vi "Write Calibration File.vi"(6 "CalDataIn":T1(array[cluster]) {"ChlFactor" format="%.3f"; "ChlZero" format="%.3f"}, 7 "CalFilepath":path) -> ()   [LabVIEW 2013]
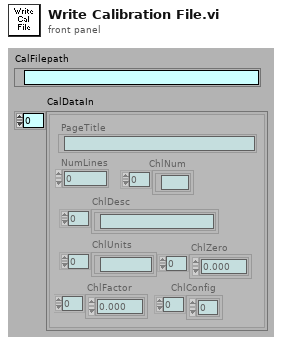
[diagram p1: front panel]
types:
  T1 = cluster{"PageTitle":string, "NumLines":i32, "ChlNum":string[], "ChlDesc":string[], "ChlUnits":string[], "ChlZero":sgl[], "ChlFactor":sgl[], "ChlConfig":u16[]}[]
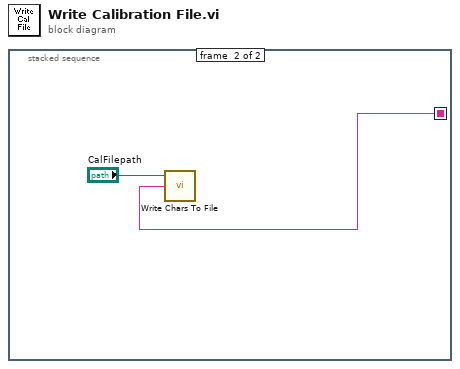
[diagram p0: block diagram]
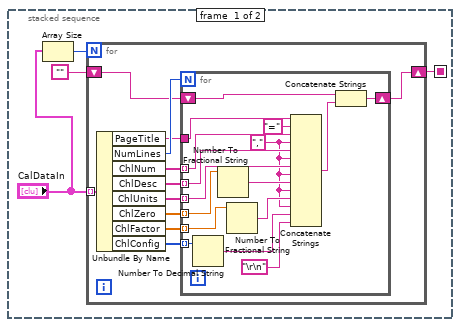
[diagram p2: hidden frame]
diagram:
  n1 = stacked-sequence {
    seq-local: [w2 _] -> [_ w32]
    frame #0 {
      n2 = Array Size(array="CalDataIn") -> (size(s)=w4:i32)
      n3 = for {
        N: w4 -> [_]
        tunnel: "CalDataIn" -> [w15] mode=indexing
        shift-right: [w5] -> w2
        shift-left: "" -> [w6]
        n4 = Unbundle By Name(w15) -> ("PageTitle"=w13:string, "NumLines"=w14:i32, "ChlNum"=w12:string[], "ChlDesc"=w11:string[], "ChlUnits"=w10:string[], "ChlZero"=w9:sgl[], "ChlFactor"=w8:sgl[], "ChlConfig"=w7:u16[])
        n5 = for {
          N: w14 -> [_]
          tunnel: w13 -> [w31]
          tunnel: w12 -> [w29] mode=indexing
          tunnel: w11 -> [w28] mode=indexing
          tunnel: w10 -> [w27] mode=indexing
          tunnel: w9 -> [w26] mode=indexing
          tunnel: w8 -> [w24] mode=indexing
          tunnel: w7 -> [w21] mode=indexing
          shift-right: [w18] -> w5
          shift-left: w6 -> [w17]
          w22 = "," ("Substring")
          n6 = Number To Decimal String(number=w21) -> (decimal integer string=w20:string)  [unwired: 1 in]
          n7 = Number To Fractional String(number=w26) -> (F-format string=w25:string)  [unwired: 3 in]
          n8 = Number To Fractional String(number=w24) -> (F-format string=w23:string)  [unwired: 3 in]
          n9 = Concatenate Strings(w31, "=" ("Substring"), w29, w22, w28, w22, w27, w22, w25, w22, w23, w22, w20, "\r\n") -> (w16:string)
          n10 = Concatenate Strings(w17, w16) -> (w18:string)
        }
      }
    }
    frame #1 {
      n11 = call "Write Chars To File.vi"("character string"=w32, "file path (dialog if empty)"="CalFilepath") -> ()  [unwired: 3 in, 1 out]
    }
  }
